vi "GetAutoRoutine.vi"(2 "Test":bool, 3 "FieldState":T10, 4 "Default Auto Routine":u16(ring), 5 "AvailableRoutines":T11) -> (0 "Selected Routine":T1[](array[typedef]) {"ArmPath"."ExtendTrajectory"."Time (ms)" items=["TrajectoryDuration_0ms"=0, "TrajectoryDuration_5ms"=5, "TrajectoryDuration_10ms"=10, "TrajectoryDuration_20ms"=20, "TrajectoryDuration_30ms"=30, "TrajectoryDuration_40ms"=40, "TrajectoryDuration_50ms"=50, "TrajectoryDuration_100ms"=100]; "ArmPath"."RotateTrajectory"."Time (ms)" items=["TrajectoryDuration_0ms"=0, "TrajectoryDuration_5ms"=5, "TrajectoryDuration_10ms"=10, "TrajectoryDuration_20ms"=20, "TrajectoryDuration_30ms"=30, "TrajectoryDuration_40ms"=40, "TrajectoryDuration_50ms"=50, "TrajectoryDuration_100ms"=100]}, 1 "Selected Routine Name":string)   [LabVIEW 2017]
uses:
  Autonomous/TypeDef/AutoRoutineSet.ctl
  Autonomous/TypeDef/AutoFieldState.ctl
  Autonomous/TypeDef/AutoPreProcessedStep.ctl
  Autonomous/PathPlannerSupport/TypeDefs/DrivePlanResponse.ctl
  Pathfinder/Pathfinder-LabVIEW/Pathfinder-Lib/VIs/Segment.ctl
  Implements/Arm/TypeDefs/ArmPlanResponse.ctl
  General/MotionProfiling/TypeDefs/TrajectoryPoint.ctl
  <vilib>/Rock Robotics/WPI/ThirdParty/Phoenix-LabVIEW/Motor Controller/Controls/CTRE_Phoenix_MotorControl_TrajectoryPointTimeDur.ctl
  Autonomous/TypeDef/AutoWaypointType.ctl
  Implements/Arm/TypeDefs/ArmTargetPosition.ctl
  Implements/TypeDefs/IntakeState.ctl
  Pathfinder/Pathfinder-LabVIEW/Pathfinder-Lib/Pathfinder.lvlib
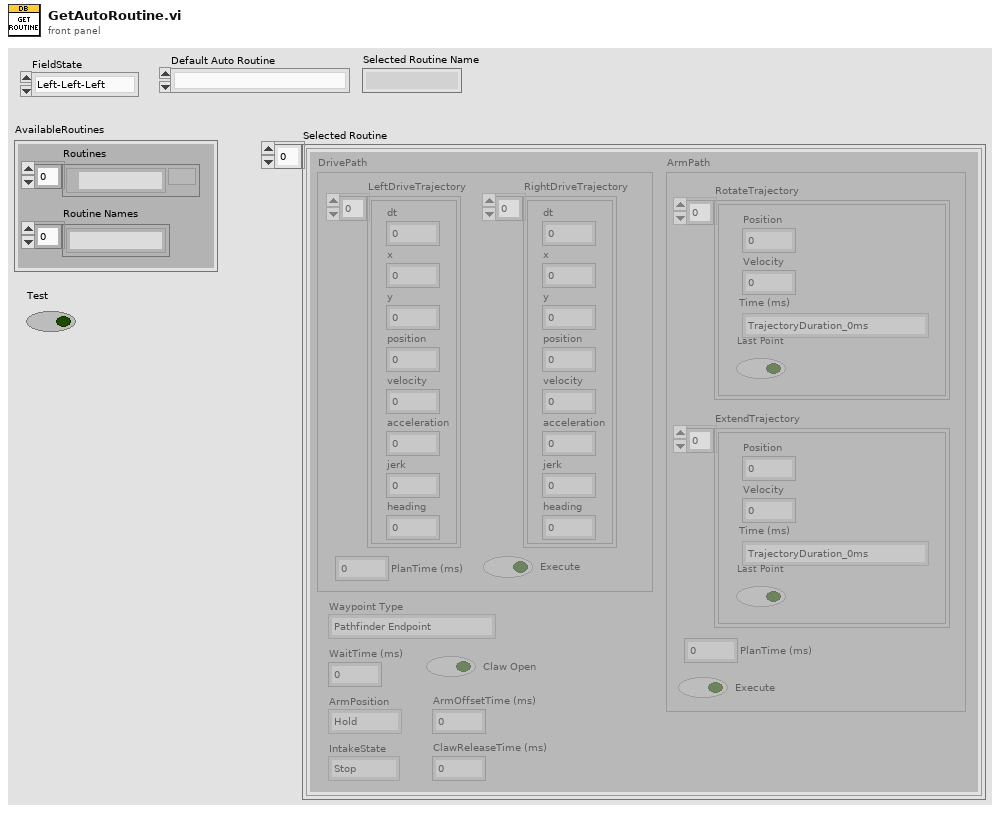
[diagram p1: front panel]
types:
  T1 = typedef "AutoPreProcessedStep.ctl" = cluster{"DrivePath":T2, "ArmPath":T4, "Waypoint Type":T7, "WaitTime (ms)":u16, "ArmPosition":T8, "IntakeState":T9, "Claw Open":bool, "ArmOffsetTime (ms)":u16, "ClawReleaseTime (ms)":i32}
  T2 = typedef "DrivePlanResponse.ctl" = cluster{"LeftDriveTrajectory":T3[], "RightDriveTrajectory":T3[], "PlanTime (ms)":u32, "Execute":bool}
  T3 = typedef "Pathfinder.lvlib/Segment.ctl" = cluster{"dt":dbl, "x":dbl, "y":dbl, "position":dbl, "velocity":dbl, "acceleration":dbl, "jerk":dbl, "heading":dbl}
  T4 = typedef "ArmPlanResponse.ctl" = cluster{"RotateTrajectory":T5[], "ExtendTrajectory":T5[], "PlanTime (ms)":u32, "Execute":bool}
  T5 = typedef "TrajectoryPoint.ctl" = cluster{"Position ":dbl, "Velocity ":dbl, "Time (ms)":T6, "Last Point":bool}
  T6 = typedef "CTRE_Phoenix_MotorControl_TrajectoryPointTimeDur.ctl" = i32
  T7 = typedef "AutoWaypointType.ctl" = enum16{"Pathfinder Endpoint", "Pathfinder Waypoint", "Zero-Radius Turn Endpoint", "Stationary", "Vision Assist Endpoint", "Stop"}
  T8 = typedef "ArmTargetPosition.ctl" = enum16{"Hold", "Switch", "Scale Low", "Scale High", "Climb", "Back Place"}
  T9 = typedef "IntakeState.ctl" = enum16{"Stop", "Forward", "Reverse", "Forward Open"}
  T10 = typedef "AutoFieldState.ctl" = enum16{"Left-Left-Left", "Left-Right-Left", "Right-Left-Right", "Right-Right-Right", "Unknown"}
  T11 = typedef "AutoRoutineSet.ctl" = cluster{"Routine Names":string[], "Routines":path[]}
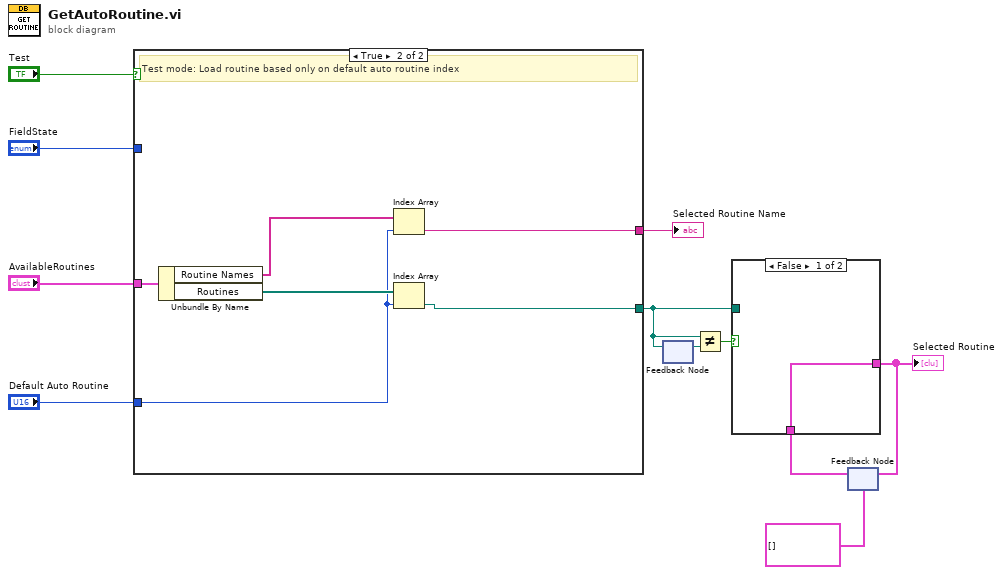
[diagram p0: block diagram]
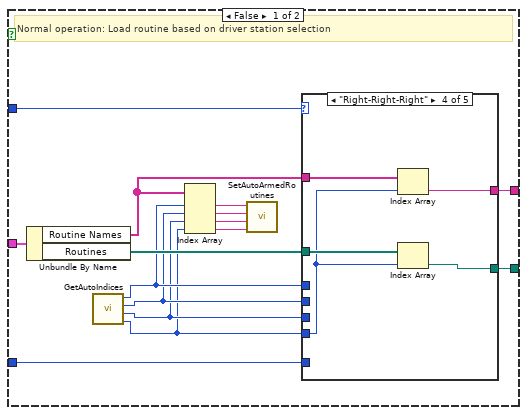
[diagram p2: hidden frame]
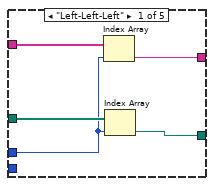
[diagram p3: hidden frame]
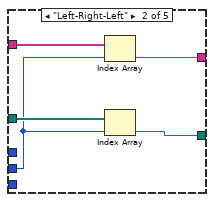
[diagram p4: hidden frame]
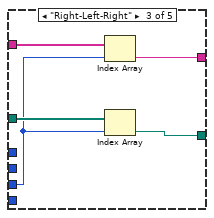
[diagram p5: hidden frame]
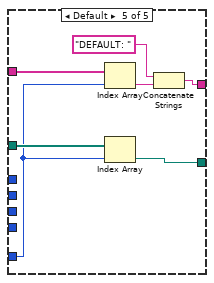
[diagram p6: hidden frame]
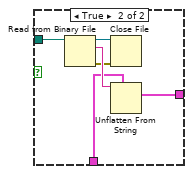
[diagram p7: hidden frame]
diagram:
  n1 = case shown="True" "Test" {
    tunnel: "FieldState" -> [w26 _]
    tunnel: "AvailableRoutines" -> [w25 w59]
    tunnel: "Default Auto Routine" -> [w23 w54]
    tunnel: [w22 w56] -> w8
    tunnel: [w12 w55] -> w3
    frame False {
      # "Normal operation: Load routine based on driver station selection"
      n2 = Unbundle By Name(w25) -> ("Routine Names"=w21:string[], "Routines"=w24:path[])
      n3 = call "GetAutoIndices.vi"() -> ("LLL Routine Index"=w20:u16, "LRL Routine Index"=w19:u16, "RLR Routine Index"=w18:u16, "RRR Routine Index"=w17:u16)  [unwired: 1 in]
      n4 = Index Array(array=w21, index #1=w20, index #2=w19, index #3=w18, index #4=w17) -> (element #1=w16:string, element #2=w15:string, element #3=w14:string, element #4=w13:string)
      n5 = call "SetAutoArmedRoutines.vi"("Routine_RRR"=w13, "Routine_RLR"=w14, "Routine_LRL"=w15, "Routine_LLL"=w16) -> ()  [unwired: 1 in]
      n6 = case shown="\"Right-Right-Right\"" w26 {
        tunnel: w24 -> [w31 w36 w41 w46 w53]
        tunnel: w20 -> [w28 _ _ _ _]
        tunnel: w19 -> [_ w33 _ _ _]
        tunnel: w18 -> [_ _ w37 _ _]
        tunnel: w17 -> [_ _ _ w42 _]
        tunnel: w23 -> [_ _ _ _ w50]
        tunnel: [w30 w35 w40 w45 w52] -> w12
        tunnel: w21 -> [w29 w34 w38 w43 w51]
        tunnel: [w27 w32 w39 w44 w47] -> w22
        frame "Left-Left-Left" {
          n7 = Index Array(array=w29, index=w28) -> (element=w27:string)
          n8 = Index Array(array=w31, index=w28) -> (element=w30:path)
        }
        frame "Left-Right-Left" {
          n9 = Index Array(array=w34, index=w33) -> (element=w32:string)
          n10 = Index Array(array=w36, index=w33) -> (element=w35:path)
        }
        frame "Right-Left-Right" {
          n11 = Index Array(array=w38, index=w37) -> (element=w39:string)
          n12 = Index Array(array=w41, index=w37) -> (element=w40:path)
        }
        frame "Right-Right-Right" {
          n13 = Index Array(array=w43, index=w42) -> (element=w44:string)
          n14 = Index Array(array=w46, index=w42) -> (element=w45:path)
        }
        frame Default {
          n15 = Index Array(array=w51, index=w50) -> (element=w49:string)
          n16 = Index Array(array=w53, index=w50) -> (element=w52:path)
          n17 = Concatenate Strings("DEFAULT: " ("string"), w49) -> (w47:string)
        }
      }
    }
    frame True {
      # "Test mode: Load routine based only on default auto routine index"
      n18 = Unbundle By Name(w59) -> ("Routine Names"=w58:string[], "Routines"=w57:path[])
      n19 = Index Array(array=w58, index=w54) -> (element=w56:string)
      n20 = Index Array(array=w57, index=w54) -> (element=w55:path)
    }
  }
  "Selected Routine Name" <- w8
  n21 = feedback-in #1(w3) -> ()
  n22 = feedback #1() -> (w7:path)  [unwired: 1 in]
  n23 = Not Equal?(x=w3, y=w7) -> (x != y?=w4:bool)
  n24 = feedback #2(T1[] [] ("Selected Routine")) -> (w5:T1[])
  n25 = case shown="False" w4 {
    tunnel: w5 -> [w60 w64]
    tunnel: [w60 w61] -> w2
    tunnel: w3 -> [_ w66]
    frame False {
    }
    frame True {
      n26 = Read from Binary File(11:w66) -> (0:w63:errorcluster, 2:w65:string, 3:w62:refnum<file>)  [unwired: 5 in, 1 out]
      n27 = Close File(refnum=w62, error in=w63) -> ()  [unwired: 2 out]
      n28 = Unflatten From String(type=w64, binary string=w65) -> (value=w61:T1[])  [unwired: 3 in, 2 out]
    }
  }
  "Selected Routine" <- w2
  n29 = feedback-in #2(w2) -> ()
